vi "Read Point CP CV Sweep.vi"(8 "error in":errorcluster, 10 "Numeric":u64, 11 "Set Point for\nCV CV Sweep":i64[](array[numeric])) -> (0 "error Out":errorcluster, 1 "Last Number":u64, 2 "Ind":bool, 4 "CP CV Ind":bool[](array[boolean]), 5 "CP CV Read Point":u64[](array[numeric]))   [LabVIEW 2012]
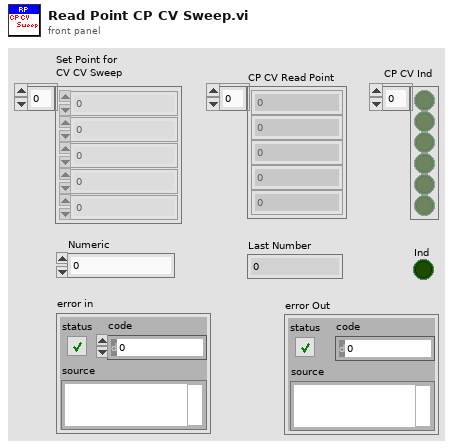
[diagram p1: front panel]
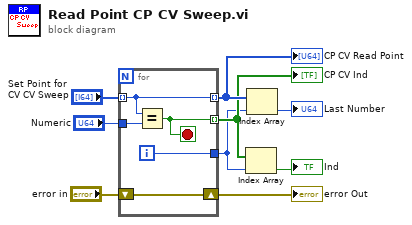
[diagram p0: block diagram]
diagram:
  n1 = for {
    tunnel: "Set Point for\nCV CV Sweep" -> [w13] mode=indexing
    tunnel: "Numeric" -> [w14]
    tunnel: [w13] -> w7 mode=indexing
    tunnel: [w12] -> w5 mode=indexing
    tunnel: [w11] -> w4
    shift-right: [w10] -> w1
    shift-left: "error in" -> [w10]
    i -> [w11]
    stop <- w12 stop-if-true
    n2 = Equal?(x=w13, y=w14) -> (x = y?=w12:bool)
  }
  "CP CV Read Point" <- w7
  "CP CV Ind" <- w5
  "error Out" <- w1
  n3 = Index Array(array=w5, index=w4) -> (element=→"Ind":bool)
  n4 = Index Array(array=w7, index=w4) -> (element=→"Last Number":i64)
